vi "Tempo prova hhmmss.vi"(11 "Tempo [s]":dbl) -> (3 "H:m:s":string)   [LabVIEW 2019]
panel:
  out "ore":dbl
  out "minuti":dbl
  out "secondi":dbl
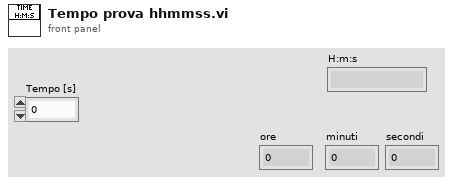
[diagram p1: front panel]
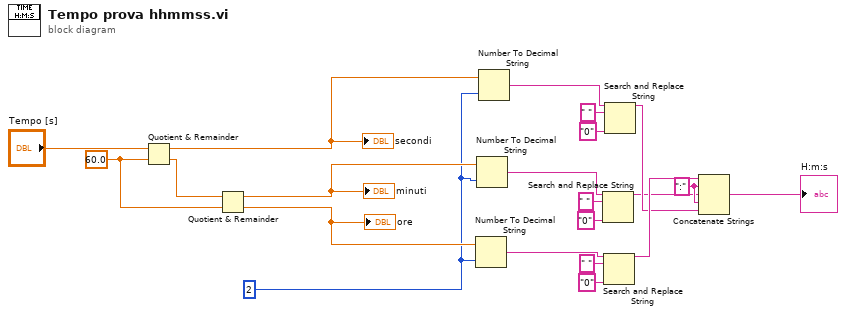
[diagram p0: block diagram]
diagram:
  w1 = 2
  w15 = ":" ("string")
  w19 = 60.0 ("y")
  n1 = Quotient & Remainder(x="Tempo [s]", y=w19) -> (x-y*floor(x/y)=w18:dbl, floor(x/y)=w20:dbl)
  "secondi" <- w18
  n2 = Quotient & Remainder(x=w20, y=w19) -> (x-y*floor(x/y)=w17:dbl, floor(x/y)=w16:dbl)
  "minuti" <- w17
  "ore" <- w16
  n3 = Number To Decimal String(number=w16, width (-)=w1) -> (decimal integer string=w13:string)
  n4 = Number To Decimal String(number=w17, width (-)=w1) -> (decimal integer string=w3:string)
  n5 = Number To Decimal String(number=w18, width (-)=w1) -> (decimal integer string=w5:string)
  n6 = Search and Replace String(input string=w3, search string=" ", replace string="0" ("replace string (\"\")")) -> (result string=w2:string)  [unwired: 5 in, 3 out]
  n7 = Search and Replace String(input string=w13, search string=" ", replace string="0" ("replace string (\"\")")) -> (result string=w10:string)  [unwired: 5 in, 3 out]
  n8 = Search and Replace String(input string=w5, search string=" ", replace string="0" ("replace string (\"\")")) -> (result string=w4:string)  [unwired: 5 in, 3 out]
  n9 = Concatenate Strings(w10, w15, w2, w15, w4) -> (→"H:m:s":string)
